vi "DateTimeToStringDateWith0.vi"(10 "time stamp":timestamp format="%<%H:%M\n%x>T") -> (0 "Dateyyyymmdd":string, 2 "String Date With0":string)   [LabVIEW 2012]
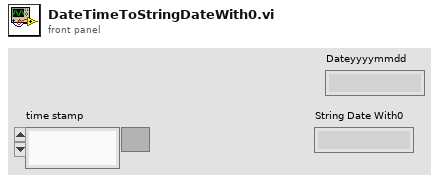
[diagram p1: front panel]
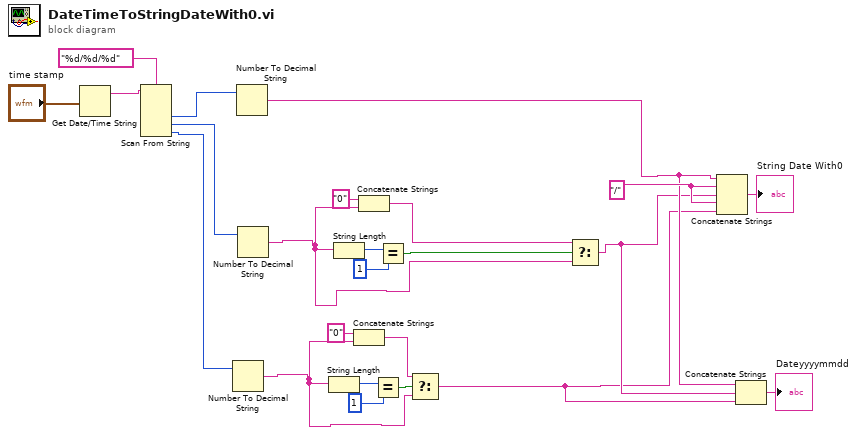
[diagram p0: block diagram]
diagram:
  w7 = "/" ("string")
  n1 = Get Date/Time String(seconds (now)="time stamp") -> (date string=w24:string)  [unwired: 2 in, 1 out]
  n2 = Scan From String(format string="%d/%d/%d", input string=w24) -> (output 1=w22:i32, output 2=w9:i32, output 3=w8:i32)  [unwired: 5 in, 3 out]
  n3 = Number To Decimal String(number=w8) -> (decimal integer string=w10:string)  [unwired: 1 in]
  n4 = Number To Decimal String(number=w22) -> (decimal integer string=w4:string)  [unwired: 1 in]
  n5 = Number To Decimal String(number=w9) -> (decimal integer string=w16:string)  [unwired: 1 in]
  n6 = String Length(string=w10) -> (length=w15:i32)
  n7 = String Length(string=w16) -> (length=w21:i32)
  n8 = Concatenate Strings("0" ("string"), w10) -> (w11:string)
  n9 = Concatenate Strings("0" ("string"), w16) -> (w17:string)
  n10 = Equal?(x=w15, y=1) -> (x = y?=w13:bool)
  n11 = Equal?(x=w21, y=1) -> (x = y?=w19:bool)
  n12 = Select(t=w11, s=w13, f=w10) -> (s? t:f=w2:string)
  n13 = Select(t=w17, s=w19, f=w16) -> (s? t:f=w3:string)
  n14 = Concatenate Strings(w4, w7, w3, w7, w2) -> (→"String Date With0":string)
  n15 = Concatenate Strings(w4, w3, w2) -> (→"Dateyyyymmdd":string)
